vi "Send Remote Request.vi"(5 "Target Task (None)":string, 6 "Timeout mS (5000)":i32=5000, 7 "Target Name":string, 8 "error in (no error)":errorcluster, 9 "Message Type":string, 10 "Message":refnum<class "Message.lvclass">, 11 "VolatusAPI in":refnum<class "VolatusAPI.lvclass">) -> (0 "error out":errorcluster, 2 "Reply":T1, 3 "VolatusAPI out":refnum<class "VolatusAPI.lvclass">)   [LabVIEW 2020, in "Volatus.lvlib" / "VolatusAPI.lvclass"]
uses:
  VolatusAPI.lvclass
  lv-protoc/LV-Proto/Message/Message.lvclass
  lv-vecto/Vecto/proto/TcpPayload/Data.ctl
  VolatusAPI.lvclass/VolatusAPI.ctl
  lv-vecto/Vecto/TCPMessageService/TCPMessageAPI.lvclass
  lv-vecto/Vecto/proto/TcpPayload/TcpPayload.lvlib
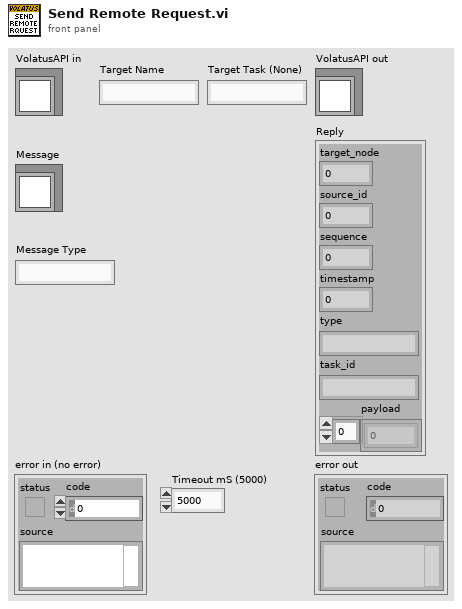
[diagram p1: front panel]
types:
  T1 = typedef "TcpPayload.lvlib/Data.ctl" = cluster{"target_node":u32, "source_id":u32, "sequence":u32, "timestamp":i64, "type":string, "task_id":string, "payload":u8[]}
  T2 = typedef "VolatusConfig.lvlib/Target Info.ctl" = cluster{"ID":u32, "Type":T3}
  T3 = typedef "VolatusConfig.lvlib/Target Type.ctl" = enum16{"Unknown", "Node", "Group"}
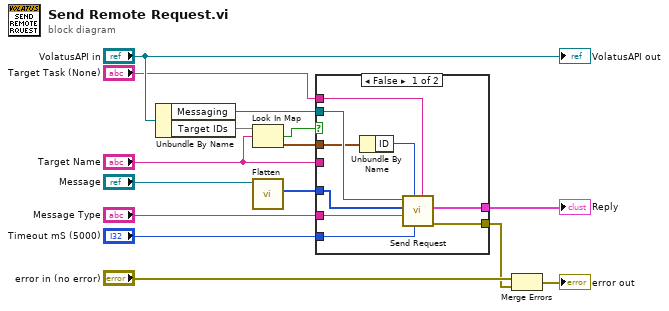
[diagram p0: block diagram]
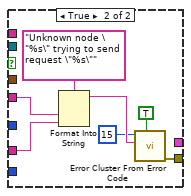
[diagram p2: hidden frame]
diagram:
  n1 = Unbundle By Name("VolatusAPI in") -> ("Messaging"=w13:refnum<class "TCPMessageAPI.lvclass">, "Target IDs"=w12:map{string, T2})
  n2 = Look In Map(map=w12, key="Target Name") -> (key not found?=w8:bool, value=w11:T2)  [unwired: 1 in]
  n3 = call-dynamic "Flatten.vi"("Message in"="Message") -> ("Buffer"=w4:u8[])  [unwired: 8 in, 2 out]
  n4 = case shown="False" w8 {
    tunnel: w13 -> [w24 _]
    tunnel: w11 -> [w17 _]
    tunnel: "Timeout mS (5000)" -> [w23 _]
    tunnel: "Target Task (None)" -> [w22 _]
    tunnel: "Target Name" -> [_ w30]
    tunnel: "Message Type" -> [w21 w29]
    tunnel: w4 -> [w20 _]
    tunnel: [w19 w28] -> w1
    tunnel: [w18 _] -> w2
    frame False {
      n5 = Unbundle By Name(w17) -> ("ID"=w16:u32)
      n6 = call "Send Request.vi"("Target Task"=w22, "Timeout mS (5000)"=w23, "Target Node"=w16, "Type"=w21, "Payload"=w20, "TCPMessageAPI in"=w24) -> ("error out"=w19:errorcluster, "Reply"=w18:T1)  [unwired: 3 in, 1 out]
    }
    frame True {
      n7 = Format Into String(format string="Unknown node \"%s\" trying to send request \"%s\"", w30, w29) -> (resulting string=w26:string)  [unwired: 2 in, 1 out]
      n8 = call <vilib>:"Error Cluster From Error Code.vi"("show call chain? (False)"=TRUE, "error message (\"\")"=w26, "error code (0)"=15) -> ("error out"=w28:errorcluster)  [unwired: 6 in]
    }
  }
  "Reply" <- w2
  n9 = Merge Errors("error in (no error)", w1) -> (→"error out":errorcluster)
  "VolatusAPI out" <- "VolatusAPI in"
